vi "9207 16Ch Analog Input.vi"(1 "9207 I/O":T1={"9207 AI0"="NI 9207/AI0", "9207 AI1"="NI 9207/AI1", "9207 AI2"="NI 9207/AI2", "9207 AI3"="NI 9207/AI3", "9207 AI4"="NI 9207/AI4", "9207 AI5"="NI 9207/AI5", "9207 AI6"="NI 9207/AI6", "9207 AI7"="NI 9207/AI7", "9207 AI8"="NI 9207/AI8", "9207 AI9"="NI 9207/AI9", "9207 AI10"="NI 9207/AI10", "9207 AI11"="NI 9207/AI11", "9207 AI12"="NI 9207/AI12", "9207 AI13"="NI 9207/AI13", "9207 AI14"="NI 9207/AI14", "9207 AI15"="NI 9207/AI15"}) -> (0 "Packets":u64[](array[numeric]))   [LabVIEW 2010]
uses:
  <vilib>/eio/EIONode/EIONode.xnode
  <vilib>/rvi/eio/nirviEIOImplementation/nirviEIOImplementation.xnode
  <vilib>/rvi/eio/common/nirviEmuClasses.ctl
  <vilib>/rvi/eio/common/nirviEmuTemplateMethod_noerrors.vi
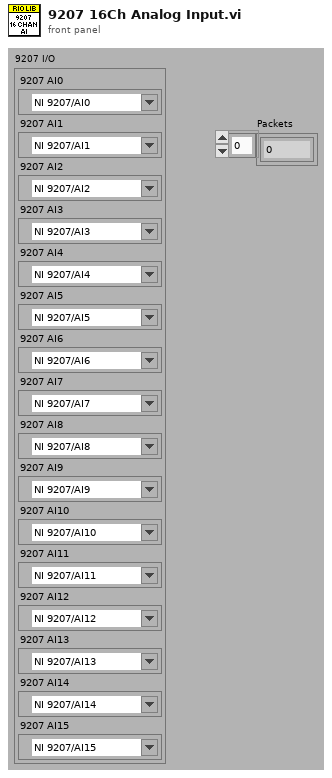
[diagram p1: front panel]
types:
  T1 = cluster{"9207 AI0":refnum<k21>, "9207 AI1":refnum<k21>, "9207 AI2":refnum<k21>, "9207 AI3":refnum<k21>, "9207 AI4":refnum<k21>, "9207 AI5":refnum<k21>, "9207 AI6":refnum<k21>, "9207 AI7":refnum<k21>, "9207 AI8":refnum<k21>, "9207 AI9":refnum<k21>, "9207 AI10":refnum<k21>, "9207 AI11":refnum<k21>, "9207 AI12":refnum<k21>, "9207 AI13":refnum<k21>, "9207 AI14":refnum<k21>, "9207 AI15":refnum<k21>}
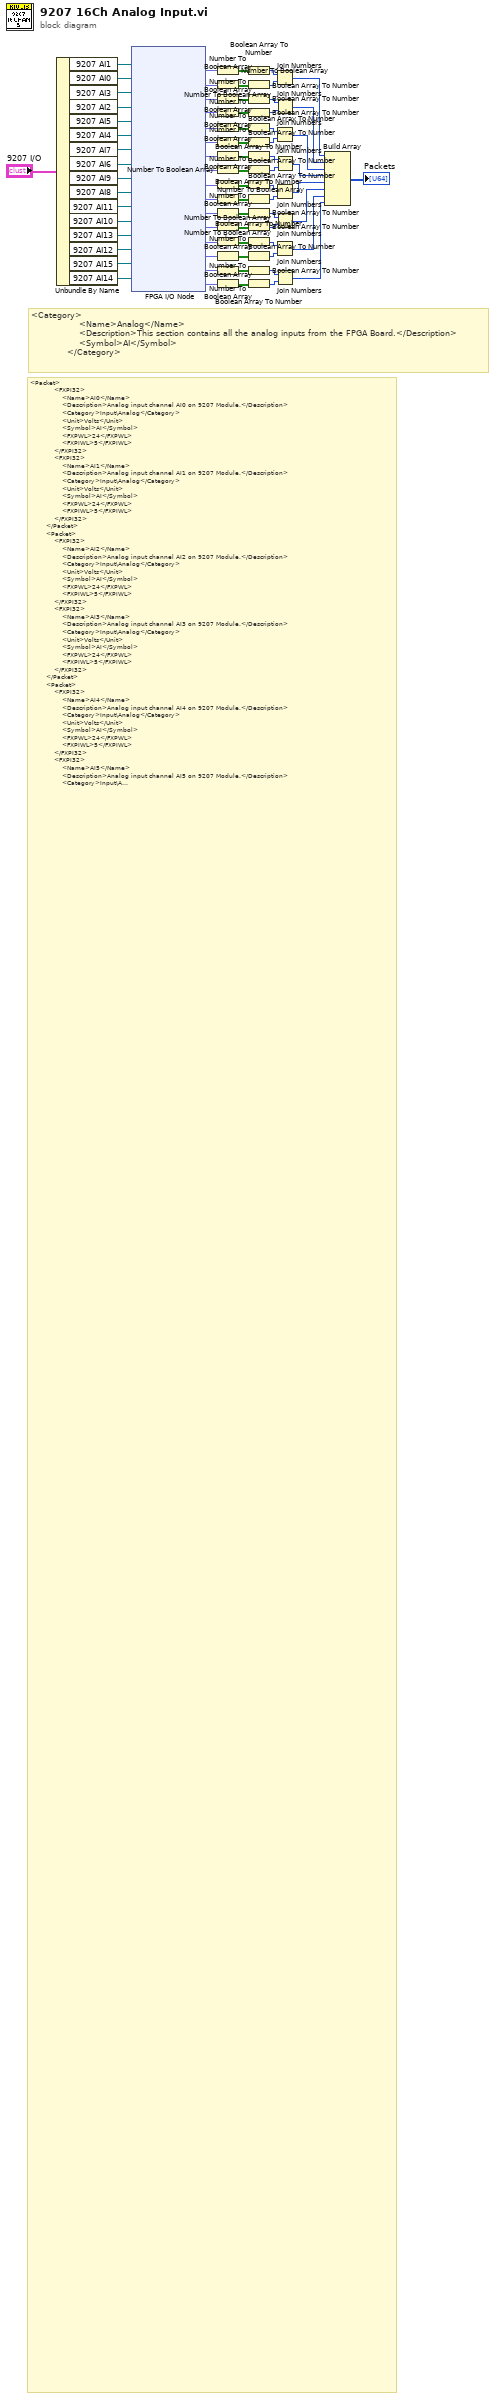
[diagram p0: block diagram]
diagram:
  # "<Category>\n                <Name>Analog</Name>\n                <Description>This section contains all the analog inputs from the FPGA Board.</Description>\n                <Symbol>AI</Symbol>\n            </Category>"
  # "<Packet>\n            <FXPI32>\n                <Name>AI0</Name>\n                <Description>Analog input channel AI0 on 9207 Module.</Description>\n                <Category>Input\\Analog</Category>\n                <Unit>Volts</Unit>\n                <Symbol>AI</Symbol>\n                <FXPWL>24</FXPWL>\n                <FXPIWL>5</FXPIWL>\n            </FXPI32>\n            <FXPI32>\n                <Name>AI1</Name>\n                <Description>Analog input channel AI1 on 9207 Module.</Description>\n                <Category>Input\\Analog</Category>\n                <Unit>Volts</Unit>\n                <Symbol>AI</Symbol>\n                <FXPWL>24</FXPWL>\n                <FXPIWL>5</FXPIWL>\n            </FXPI32>\n        </Packet>\n        <Packet>\n            <FXPI32>\n                <Name>AI2</Name>\n                <Description>Analog input channel AI2 on 9207 Module.</Description>\n                <Category>Input\\Analog</Category>\n                <Unit>Volts</Unit>\n                <Symbol>AI</Symbol>\n                <FXPWL>24</FXPWL>\n                <FXPIWL>5</FXPIWL>\n            </FXPI32>\n            <FXPI32>\n                <Name>AI3</Name>\n                <Description>Analog input channel AI3 on 9207 Module.</Description>\n                <Category>Input\\Analog</Category>\n                <Unit>Volts</Unit>\n                <Symbol>AI</Symbol>\n                <FXPWL>24</FXPWL>\n                <FXPIWL>5</FXPIWL>\n            </FXPI32>\n        </Packet>\n        <Packet>\n            <FXPI32>\n                <Name>AI4</Name>\n                <Description>Analog input channel AI4 on 9207 Module.</Description>\n                <Category>Input\\Analog</Category>\n                <Unit>Volts</Unit>\n                <Symbol>AI</Symbol>\n                <FXPWL>24</FXPWL>\n                <FXPIWL>5</FXPIWL>\n            </FXPI32>\n            <FXPI32>\n                <Name>AI5</Name>\n                <Description>Analog input channel AI5 on 9207 Module.</Description>\n                <Category>Input\\Analog</Category>\n                <Unit>Volts</Unit>\n                <Symbol>AI</Symbol>\n                <FXPWL>24</FXPWL>\n                <FXPIWL>5</FXPIWL>\n            </FXPI32>\n        </Packet>\n        <Packet>\n            <FXPI32>\n                <Name>AI6</Name>\n                <Description>Analog input channel AI6 on 9207 Module.</Description>\n                <Category>Input\\Analog</Category>\n                <Unit>Volts</Unit>\n                <Symbol>AI</Symbol>\n                <FXPWL>24</FXPWL>\n                <FXPIWL>5</FXPIWL>\n            </FXPI32>\n            <FXPI32>\n                <Name>AI7</Name>\n                <Description>Analog input channel AI7 on 9207 Module.</Description>\n                <Category>Input\\Analog</Category>\n                <Unit>Volts</Unit>\n                <Symbol>AI</Symbol>\n                <FXPWL>24</FXPWL>\n                <FXPIWL>5</FXPIWL>\n            </FXPI32>\n        </Packet>\n        <Packet>\n            <FXPI32>\n                <Name>AI8</Name>\n                <Description>Analog input channel AI8 on 9207 Module.</Description>\n                <Category>Input\\Analog</Category>\n                <Unit>Amps</Unit>\n                <Symbol>AI</Symbol>\n                <FXPWL>24</FXPWL>\n                <FXPIWL>-4</FXPIWL>\n            </FXPI32>\n            <FXPI32>\n                <Name>AI9</Name>\n                <Description>Analog input channel AI9 on 9207 Module.</Description>\n                <Category>Input\\Analog</Category>\n                <Unit>Amps</Unit>\n                <Symbol>AI</Symbol>\n                <FXPWL>24</FXPWL>\n                <FXPIWL>-4</FXPIWL>\n            </FXPI32>\n        </Packet>\n        <Packet>\n            <FXPI32>\n                <Name>AI10</Name>\n                <Description>Analog input channel AI10 on 9207 Module.</Description>\n                <Category>Input\\Analog</Category>\n                <Unit>Amps</Unit>\n                <Symbol>AI</Symbol>\n                <FXPWL>24</FXPWL>\n                <FXPIWL>-4</FXPIWL>\n            </FXPI32>\n            <FXPI32>\n                <Name>AI11</Name>\n                <Description>Analog input channel AI11 on 9207 Module.</Description>\n                <Category>Input\\Analog</Category>\n                <Unit>Amps</Unit>\n                <Symbol>AI</Symbol>\n                <FXPWL>24</FXPWL>\n                <FXPIWL>-4</FXPIWL>\n            </FXPI32>\n        </Packet>\n        <Packet>\n            <FXPI32>\n                <Name>AI12</Name>\n                <Description>Analog input channel AI12 on 9207 Module.</Description>\n                <Category>Input\\Analog</Category>\n                <Unit>Amps</Unit>\n                <Symbol>AI</Symbol>\n                <FXPWL>24</FXPWL>\n                <FXPIWL>-4</FXPIWL>\n            </FXPI32>\n            <FXPI32>\n                <Name>AI13</Name>\n                <Description>Analog input channel AI13 on 9207 Module.</Description>\n                <Category>Input\\Analog</Category>\n                <Unit>Amps</Unit>\n                <Symbol>AI</Symbol>\n                <FXPWL>24</FXPWL>\n                <FXPIWL>-4</FXPIWL>\n            </FXPI32>\n        </Packet>\n        <Packet>\n            <FXPI32>\n                <Name>AI14</Name>\n                <Description>Analog input channel AI14 on 9207 Module.</Description>\n                <Category>Input\\Analog</Category>\n                <Unit>Amps</Unit>\n                <Symbol>AI</Symbol>\n                <FXPWL>24</FXPWL>\n                <FXPIWL>-4</FXPIWL>\n            </FXPI32>\n            <FXPI32>\n                <Name>AI15</Name>\n                <Description>Analog input channel AI15 on 9207 Module.</Description>\n                <Category>Input\\Analog</Category>\n                <Unit>Amps</Unit>\n                <Symbol>AI</Symbol>\n                <FXPWL>24</FXPWL>\n                <FXPIWL>-4</FXPIWL>\n            </FXPI32>\n        </Packet>"
  n1 = Unbundle By Name("9207 I/O") -> ("9207 AI1"=w64:refnum<k21>, "9207 AI0"=w65:refnum<k21>, "9207 AI3"=w66:refnum<k21>, "9207 AI2"=w59:refnum<k21>, "9207 AI5"=w58:refnum<k21>, "9207 AI4"=w47:refnum<k21>, "9207 AI7"=w48:refnum<k21>, "9207 AI6"=w49:refnum<k21>, "9207 AI9"=w50:refnum<k21>, "9207 AI8"=w51:refnum<k21>, "9207 AI11"=w52:refnum<k21>, "9207 AI10"=w53:refnum<k21>, "9207 AI13"=w54:refnum<k21>, "9207 AI12"=w55:refnum<k21>, "9207 AI15"=w56:refnum<k21>, "9207 AI14"=w57:refnum<k21>)
  n2 = xnode "FPGA I/O Node"("FPGA I/O In"=w64, "FPGA I/O In"=w65, "FPGA I/O In"=w66, "FPGA I/O In"=w59, "FPGA I/O In"=w58, "FPGA I/O In"=w47, "FPGA I/O In"=w48, "FPGA I/O In"=w49, "FPGA I/O In"=w50, "FPGA I/O In"=w51, "FPGA I/O In"=w52, "FPGA I/O In"=w53, "FPGA I/O In"=w54, "FPGA I/O In"=w55, "FPGA I/O In"=w56, "FPGA I/O In"=w57) -> ("I/O Item"=w70:fxp<+/-,24,5>, "I/O Item"=w71:fxp<+/-,24,5>, "I/O Item"=w44:fxp<+/-,24,5>, "I/O Item"=w46:fxp<+/-,24,5>, "I/O Item"=w34:fxp<+/-,24,5>, "I/O Item"=w33:fxp<+/-,24,5>, "I/O Item"=w32:fxp<+/-,24,5>, "I/O Item"=w15:fxp<+/-,24,5>, "I/O Item"=w14:fxp<+/-,24,-4>, "I/O Item"=w13:fxp<+/-,24,-4>, "I/O Item"=w12:fxp<+/-,24,-4>, "I/O Item"=w11:fxp<+/-,24,-4>, "I/O Item"=w10:fxp<+/-,24,-4>, "I/O Item"=w9:fxp<+/-,24,-4>, "I/O Item"=w8:fxp<+/-,24,-4>, "I/O Item"=w7:fxp<+/-,24,-4>)  [unwired: 16 out]
  n3 = Number To Boolean Array(number=w70) -> (Boolean array=w67:bool[])
  n4 = Number To Boolean Array(number=w71) -> (Boolean array=w68:bool[])
  n5 = Number To Boolean Array(number=w44) -> (Boolean array=w43:bool[])
  n6 = Number To Boolean Array(number=w46) -> (Boolean array=w69:bool[])
  n7 = Number To Boolean Array(number=w34) -> (Boolean array=w40:bool[])
  n8 = Number To Boolean Array(number=w33) -> (Boolean array=w39:bool[])
  n9 = Number To Boolean Array(number=w32) -> (Boolean array=w42:bool[])
  n10 = Number To Boolean Array(number=w15) -> (Boolean array=w38:bool[])
  n11 = Number To Boolean Array(number=w14) -> (Boolean array=w21:bool[])
  n12 = Number To Boolean Array(number=w13) -> (Boolean array=w20:bool[])
  n13 = Number To Boolean Array(number=w12) -> (Boolean array=w23:bool[])
  n14 = Number To Boolean Array(number=w11) -> (Boolean array=w19:bool[])
  n15 = Number To Boolean Array(number=w10) -> (Boolean array=w26:bool[])
  n16 = Number To Boolean Array(number=w9) -> (Boolean array=w27:bool[])
  n17 = Number To Boolean Array(number=w8) -> (Boolean array=w24:bool[])
  n18 = Number To Boolean Array(number=w7) -> (Boolean array=w28:bool[])
  n19 = Boolean Array To Number(Boolean array=w67) -> (number=w72:u32)
  n20 = Boolean Array To Number(Boolean array=w68) -> (number=w73:u32)
  n21 = Boolean Array To Number(Boolean array=w43) -> (number=w45:u32)
  n22 = Boolean Array To Number(Boolean array=w69) -> (number=w74:u32)
  n23 = Boolean Array To Number(Boolean array=w40) -> (number=w37:u32)
  n24 = Boolean Array To Number(Boolean array=w39) -> (number=w36:u32)
  n25 = Boolean Array To Number(Boolean array=w42) -> (number=w41:u32)
  n26 = Boolean Array To Number(Boolean array=w38) -> (number=w35:u32)
  n27 = Boolean Array To Number(Boolean array=w21) -> (number=w18:u32)
  n28 = Boolean Array To Number(Boolean array=w20) -> (number=w17:u32)
  n29 = Boolean Array To Number(Boolean array=w23) -> (number=w22:u32)
  n30 = Boolean Array To Number(Boolean array=w19) -> (number=w16:u32)
  n31 = Boolean Array To Number(Boolean array=w26) -> (number=w29:u32)
  n32 = Boolean Array To Number(Boolean array=w27) -> (number=w30:u32)
  n33 = Boolean Array To Number(Boolean array=w24) -> (number=w25:u32)
  n34 = Boolean Array To Number(Boolean array=w28) -> (number=w31:u32)
  n35 = Join Numbers(hi=w72, lo=w73) -> ((hi.lo)=w62:u64)
  n36 = Join Numbers(hi=w37, lo=w36) -> ((hi.lo)=w6:u64)
  n37 = Join Numbers(hi=w18, lo=w17) -> ((hi.lo)=w4:u64)
  n38 = Join Numbers(hi=w29, lo=w30) -> ((hi.lo)=w2:u64)
  n39 = Join Numbers(hi=w45, lo=w74) -> ((hi.lo)=w63:u64)
  n40 = Join Numbers(hi=w41, lo=w35) -> ((hi.lo)=w5:u64)
  n41 = Join Numbers(hi=w22, lo=w16) -> ((hi.lo)=w3:u64)
  n42 = Join Numbers(hi=w25, lo=w31) -> ((hi.lo)=w1:u64)
  n43 = Build Array(w62, w63, w6, w5, w4, w3, w2, w1) -> (→"Packets":u64[])
